vi "VI Tree.vi"   [LabVIEW 2025, in "TDK-Lambda GEN LAN Series.lvlib"]
doc: "Shows the LabVIEW instrument driver for the TDK-Lambda Genesys Series DC Power Supplies. The VI Tree shows all of the user-callable VIs in an organized table. \n\nThis is compatable with all TDK-Lambda Genesys Series DC Power Supplies with the LAN Option."
uses:
  <userlib>/TDK-Lambda GEN LAN Series/TDK-Lambda GEN LAN Series.lvlib
panel:
  # "(c) 2019 TDK-Lambda.  ALL RIGHTS RESERVED."
  # "SEE DIAGRAM\nFOR VI TREE."
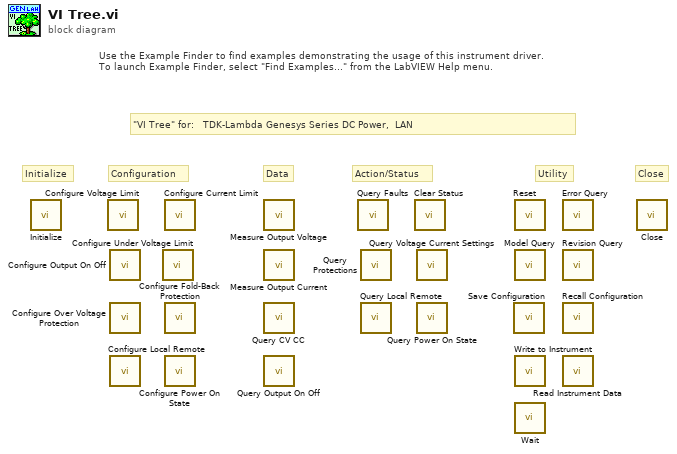
[diagram p0: block diagram]
diagram:
  # "Use the Example Finder to find examples demonstrating the usage of this instrument driver.\nTo launch Example Finder, select \"Find Examples...\" from the LabVIEW Help menu."
  # "Action/Status"
  # "Data"
  # "Utility"
  # "\"VI Tree\" for:   TDK-Lambda Genesys Series DC Power,  LAN"
  # "Configuration"
  # "Close"
  # "Initialize"
  n1 = call "Initialize.vi"() -> ()  [unwired: 10 in, 2 out]
  n2 = call <userlib>:"Configure Voltage Limit.vi"() -> ()  [unwired: 10 in, 2 out]
  n3 = call <userlib>:"Configure Output On Off.vi"() -> ()  [unwired: 10 in, 2 out]
  n4 = call <userlib>:"Configure Over Voltage Protection.vi"() -> ()  [unwired: 10 in, 2 out]
  n5 = call <userlib>:"Configure Local Remote.vi"() -> ()  [unwired: 10 in, 2 out]
  n6 = call <userlib>:"Configure Under Voltage Limit.vi"() -> ()  [unwired: 10 in, 2 out]
  n7 = call <userlib>:"Configure Current Limit.vi"() -> ()  [unwired: 10 in, 2 out]
  n8 = call <userlib>:"Configure Fold-Back Protection.vi"() -> ()  [unwired: 10 in, 2 out]
  n9 = call <userlib>:"Configure Power On State.vi"() -> ()  [unwired: 10 in, 2 out]
  n10 = call "Measure Output Voltage.vi"() -> ()  [unwired: 9 in, 3 out]
  n11 = call <userlib>:"Measure Output Current.vi"() -> ()  [unwired: 9 in, 3 out]
  n12 = call "Query CV CC.vi"() -> ()  [unwired: 6 in, 6 out]
  n13 = call "Query Output On Off.vi"() -> ()  [unwired: 9 in, 3 out]
  n14 = call <userlib>:"Query Faults.vi"() -> ()  [unwired: 7 in, 5 out]
  n15 = call <userlib>:"Query Protections.vi"() -> ()  [unwired: 7 in, 5 out]
  n16 = call <userlib>:"Query Local Remote.vi"() -> ()  [unwired: 8 in, 4 out]
  n17 = call <userlib>:"Clear Status.vi"() -> ()  [unwired: 10 in, 2 out]
  n18 = call <userlib>:"Query Voltage Current Settings.vi"() -> ()  [unwired: 8 in, 4 out]
  n19 = call <userlib>:"Query Power On State.vi"() -> ()  [unwired: 9 in, 3 out]
  n20 = call "Save Configuration.vi"() -> ()  [unwired: 10 in, 2 out]
  n21 = call "Reset.vi"() -> ()  [unwired: 10 in, 2 out]
  n22 = call "Model Query.vi"() -> ()  [unwired: 6 in, 6 out]
  n23 = call <userlib>:"Write to Instrument.vi"() -> ()  [unwired: 10 in, 2 out]
  n24 = call <userlib>:"Wait.vi"() -> ()  [unwired: 10 in, 2 out]
  n25 = call <userlib>:"Error Query.vi"() -> ()  [unwired: 8 in, 4 out]
  n26 = call "Revision Query.vi"() -> ()  [unwired: 7 in, 5 out]
  n27 = call "Recall Configuration.vi"() -> ()  [unwired: 10 in, 2 out]
  n28 = call <userlib>:"Read Instrument Data.vi"() -> ()  [unwired: 8 in, 4 out]
  n29 = call "Close.vi"() -> ()  [unwired: 11 in, 1 out]
